vi "Exemple 3_CB.vi"(4 "User Parameter":variant, 6 "Control Ref":refnum<k24>, 7 "Event Common Data":T1) -> ()   [LabVIEW 2021, in "LUGE_2022.4.lvlib"]
uses:
  C:/Users/Phalanx/Documents/LUGE/ExempleLUGE/bin/Release/ExempleLUGE.dll
  Users/Phalanx/Documents/LUGE/ExempleLUGE/bin/Release/ExempleLUGE.dll
  LUGE_2022.4.lvlib
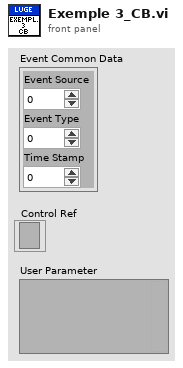
[diagram p1: front panel]
types:
  T1 = cluster{"Event Source":i32, "Event Type":u32, "Time Stamp":u32}
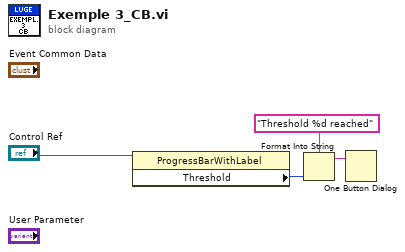
[diagram p0: block diagram]
diagram:
  n1 = property on="Property Node" class="ProgressBarWithLabel"(reference="Control Ref") -> ("Threshold"=w3:i32)  [unwired: 1 in, 2 out]
  n2 = Format Into String(format string="Threshold %d reached", w3) -> (resulting string=w1:string)  [unwired: 2 in, 1 out]
  n3 = One Button Dialog(message=w1) -> ()  [unwired: 1 in, 1 out]
